vi "Acquire Agent Public Key Refnum.vi"(8 "error in (no error)":errorcluster, 11 "agent public key":T1) -> (0 "error out":errorcluster, 2 "libssh2_agent_publickey*":u64)   [LabVIEW 2013, in "libssh2.lvlib"]
uses:
  libssh2.lvlib
  Agent Public Key Refnum.ctl
  Acquire Session.vi
  Read Agent Refnum.vi
  <vilib>/Utility/semaphor.llb/Acquire Semaphore.vi
  Read Session Refnum.vi
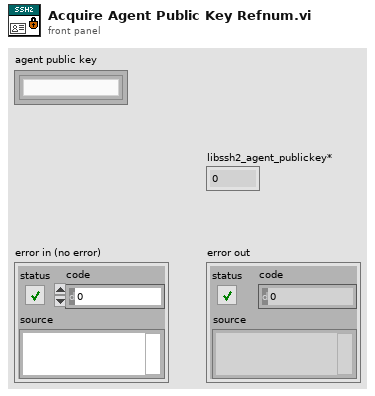
[diagram p1: front panel]
types:
  T1 = typedef "libssh2.lvlib/Agent Public Key Refnum.ctl" = refnum<k1>
  T2 = typedef "libssh2.lvlib/Agent Refnum.ctl" = refnum<k1>
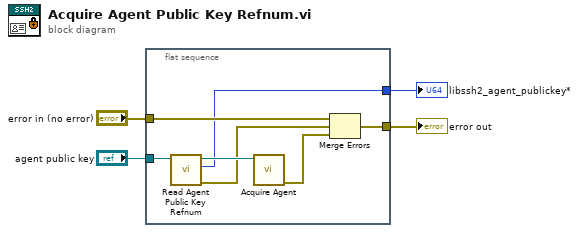
[diagram p0: block diagram]
diagram:
  n1 = flat-sequence {
    tunnel: [w8] -> w4
    tunnel: "error in (no error)" -> [w7]
    tunnel: "agent public key" -> [w6]
    tunnel: [w5] -> w1
    frame #0 {
      n2 = call "Read Agent Public Key Refnum.vi"("agent public key"=w6) -> ("error out"=w10:errorcluster, "libssh2_agent_publickey*"=w5:u64, "agent"=w11:T2)  [unwired: 8 in]
      n3 = call "Acquire Agent.vi"("agent"=w11) -> ("error out"=w9:errorcluster)  [unwired: 9 in, 1 out]
      n4 = Merge Errors(w7, w10, w9) -> (w8:errorcluster)
    }
  }
  "error out" <- w4
  "libssh2_agent_publickey*" <- w1
